vi "setUregisteredEvents.vi"(8 "error in (no error)":errorcluster, 10 "unregisteredEvents":string[](array[string]), 11 "Event.lvclass in":refnum<class "Event.lvclass">) -> (0 "error out":errorcluster, 3 "Event.lvclass out":refnum<class "Event.lvclass">)   [LabVIEW 2009, in "Events.lvlib" / "Event.lvclass"]
uses:
  Event.lvclass
  Event.lvclass/Event.ctl
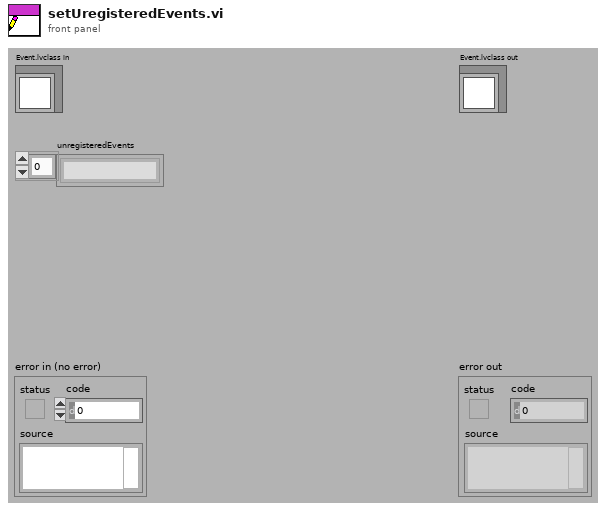
[diagram p1: front panel]
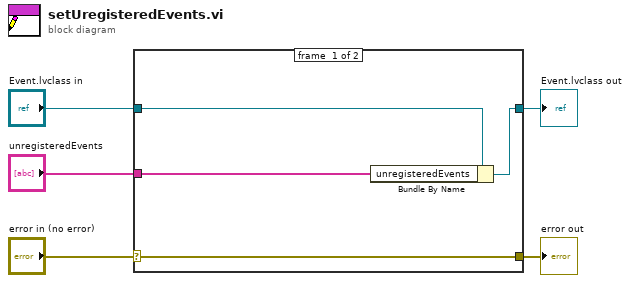
[diagram p0: block diagram]
diagram:
  n1 = case shown="No Error" "error in (no error)" {
    selector: "error in (no error)" -> [w9 w10]
    tunnel: [w9 w10] -> w4
    tunnel: [w7 w11] -> w2
    tunnel: "Event.lvclass in" -> [w8 w11]
    tunnel: "unregisteredEvents" -> [w6 _]
    frame #0 {
      n2 = Bundle By Name(cluster=w8, "unregisteredEvents"=w6) -> (w7:refnum<class "Event.lvclass">)
    }
    frame #1 {
    }
  }
  "error out" <- w4
  "Event.lvclass out" <- w2
